vi "Get Adjacent State.vi"(6 "Direction":enum16{"Previous", "Next"}(ring), 8 "error in (no error)":errorcluster, 11 "Routing Channel Page Controls":T1) -> (0 "error out":errorcluster, 3 "state name":string)   [LabVIEW 2020, in "Routing and Faulting System Explorer.lvlib"]
uses:
  Routing and Faulting System Explorer.lvlib
  Routing Channel Page Controls.ctl
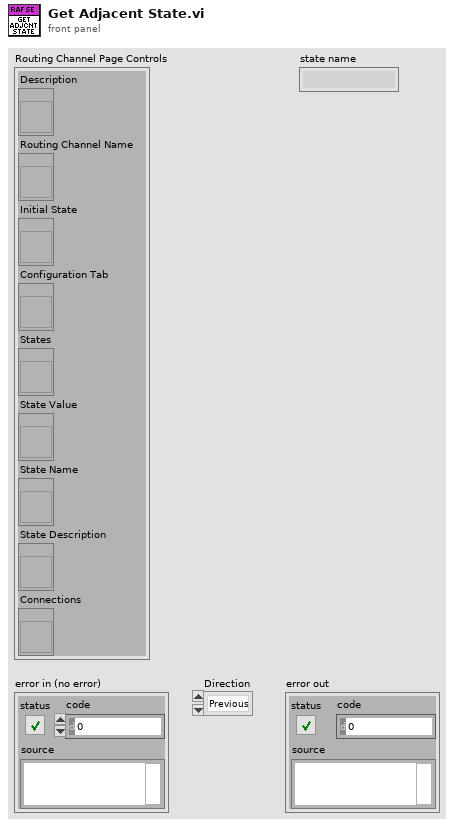
[diagram p1: front panel]
types:
  T1 = typedef "Routing and Faulting System Explorer.lvlib/Routing Channel Page Controls.ctl" = cluster{"Description":refnum<vi>, "Routing Channel Name":refnum<vi>, "Initial State":refnum<vi>, "Configuration Tab":refnum<vi>, "States":refnum<vi>, "State Value":refnum<vi>, "State Name":refnum<vi>, "State Description":refnum<vi>, "Connections":refnum<vi>}
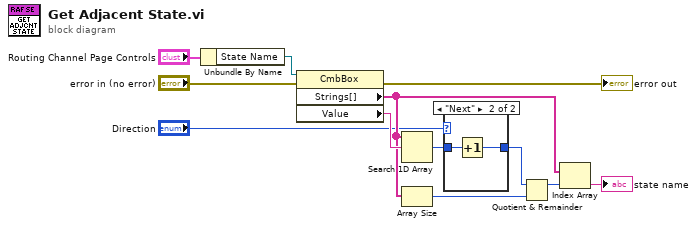
[diagram p0: block diagram]
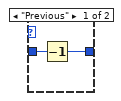
[diagram p2: hidden frame]
diagram:
  n1 = Unbundle By Name("Routing Channel Page Controls") -> ("State Name"=w11:refnum<vi>)
  n2 = property class="CmbBox"(reference=w11, error in="error in (no error)") -> (error out=→"error out":errorcluster, "Strings[]"=w6:string[], "Value"=w12:string)  [unwired: 1 out]
  n3 = Search 1D Array(1D array=w6, element=w12) -> (index of element=w2:i32)  [unwired: 1 in]
  n4 = Array Size(array=w6) -> (size(s)=w7:i32)
  n5 = case shown="\"Next\"" "Direction" {
    tunnel: w2 -> [w14 w16]
    tunnel: [w13 w15] -> w1
    frame "Previous" {
      n6 = Decrement(x=w14) -> (x-1=w13:i32)
    }
    frame "Next" {
      n7 = Increment(x=w16) -> (x+1=w15:i32)
    }
  }
  n8 = Quotient & Remainder(x=w1, y=w7) -> (x-y*floor(x/y)=w5:i32)  [unwired: 1 out]
  n9 = Index Array(array=w6, index=w5) -> (element=→"state name":string)
